vi "Main.vi"() -> ()   [LabVIEW 2014]
doc: "Use this template to build a simple state machine design pattern. Each state executes code and determines which state to transition to."
uses:
  controls/State.ctl
  controls/Data.ctl
  <vilib>/vision/Image Controls.llb/IMAQ Image.ctl
  <vilib>/userdefined/High Color/IMAQdx.ctl
panel:
  out "Tab Control":T1(tab)
  in  "Angle X":dbl(slide) scale=-90.0..90.0
  in  "Angle Y":dbl(slide) scale=-90.0..90.0
  in  "OK Button":bool
  in  "polar attributes":T2={"maximum"=1000.0, "minimum"=0.0, "clip to min"=FALSE, "log?(F)"=FALSE, "grid color"=0, "plot color"=65280, "fmt and prec"={"format"=enum."Decimal", "precision"=0}, "visible section"=8} {"minimum" format="%0.2f"; "maximum" format="%0.2f"}
  out "Image":T3(plugin-control)
  in  "Camera":refnum<k21>="cam1" caption="IMAQdx Session"
  in  "LIDAR VISA":refnum<visa-resource-name>="COM3"
  out "Data Aquired":picture
  in  "Debug Robot":bool
  in  "Reinitialize Robot":bool
  in  "Find Target":bool
  in  "Find Hole":bool
  in  "Exit":bool
  in  "Debug Angle X":dbl(slide) scale=-90.0..90.0
  in  "Debug Angle Y":dbl(slide) scale=-90.0..90.0
  in  "Debug Ok?":bool
  in  "Debug polar atributes":T2={"maximum"=300000.0, "minimum"=0.0, "clip to min"=FALSE, "log?(F)"=FALSE, "grid color"=0, "plot color"=65280, "fmt and prec"={"format"=enum."Decimal", "precision"=0}, "visible section"=8} {"minimum" format="%0.2f"; "maximum" format="%0.2f"}
  out "Debug Camera Image":T3(plugin-control)
  out "Data Aquired 2":picture
  # "Test Bench for Camera Image"
  # "Device Attributes"
  # "Select ok when all sensors and \nactuators are confirmed to be \nworking"
  # "Test Bench for Phidget Servos"
  # "Test Bench for LIDAR Data"
  # "Polar Plot Settings"
  # "Test Bench for Camera Image"
  # "Select ok when all sensors and \nactuators are confirmed to be \nworking"
  # "Test Bench for Phidget Servos"
  # "Test Bench for LIDAR Data"
  # "Polar Plot Settings"
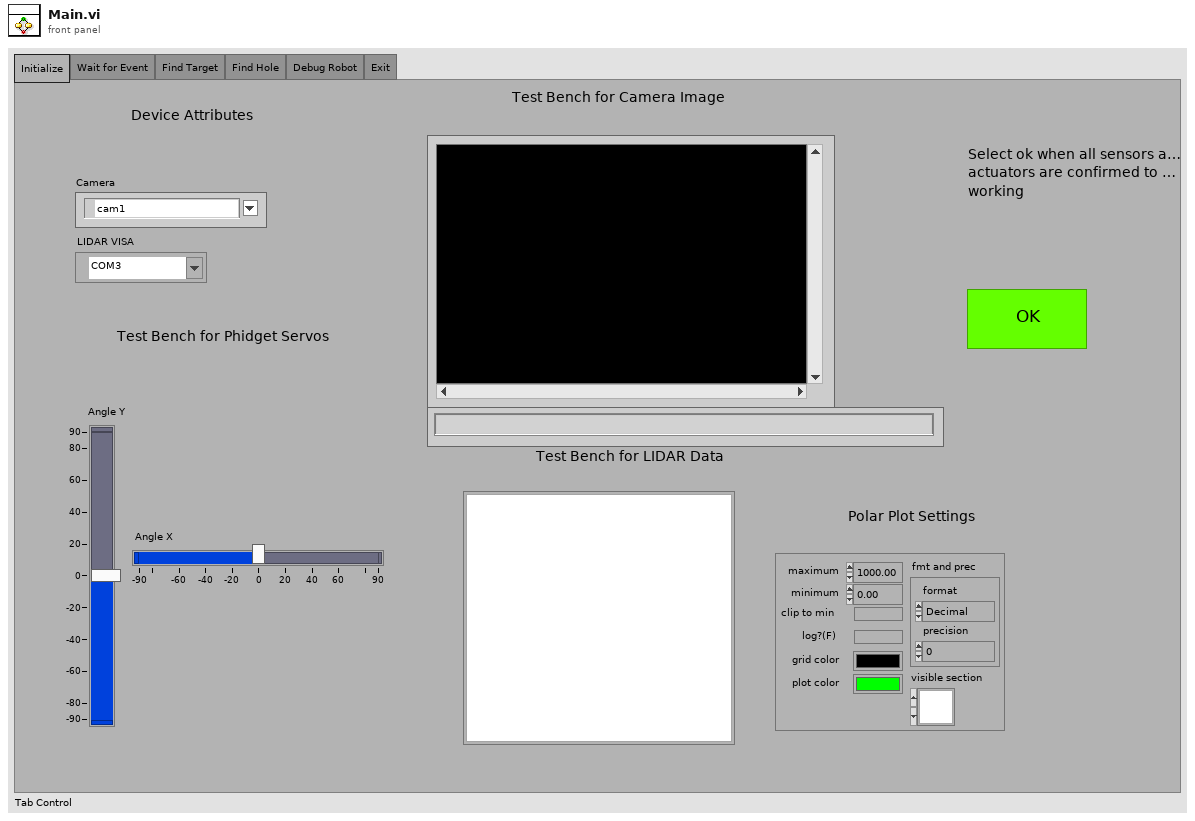
[diagram p1: front panel]
types:
  T1 = enum32{"Initialize", "Wait for Event", "Find Target", "Find Hole", "Debug Robot", "Exit"}
  T2 = cluster{"maximum":dbl, "minimum":dbl, "clip to min":bool, "log?(F)":bool, "grid color":u32, "plot color":u32, "fmt and prec":cluster{"format":enum8{"Decimal", "Scientific", "Engineering", "Binary", "Octal", "Hex"}, "precision":u8}, "visible section":u16}
  T3 = typedef "IMAQ Image.ctl" = refnum<image>
  T4 = typedef "Data.ctl" = cluster{"New Image":T3, "Session Out":T5, "LIDAR VISA Name":refnum<visa-resource-name>, "Phidget Device Out":i32, "Lidar Data":cluster{dbl, dbl}[], "polar attributes":cluster{"maximum":dbl, "minimum":dbl, "clip to min":bool, "log?(F)":bool, "grid color":u32, "plot color":u32, "fmt and prec":cluster{"format":enum8{"Decimal", "Scientific", "Engineering", "Binary", "Octal", "Hex"}, "precision":u8}, "visible section":u16}, "Debug Statement":string, "Servo Angles":cluster{"Angle X":dbl, "Angle Y":dbl}}
  T5 = typedef "IMAQdx.ctl" = refnum<k21>
  T6 = typedef "State.ctl" = enum16{"Initialize", "Wait for Event", "Find Target", "Find Hole", "Debug Robot", "Exit"}
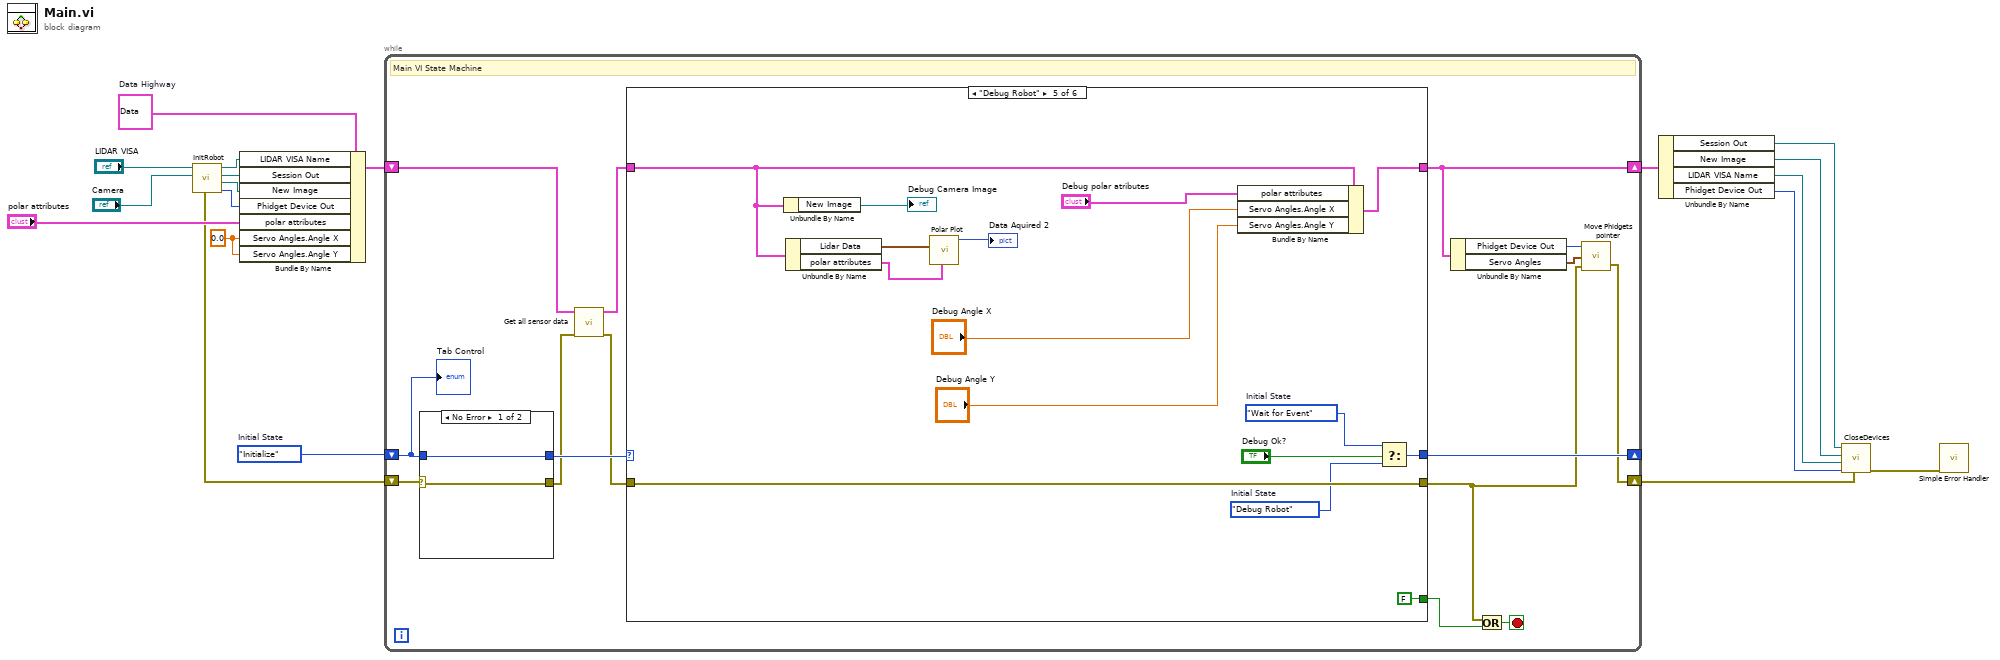
[diagram p0: block diagram]
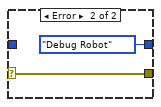
[diagram p2: hidden frame]
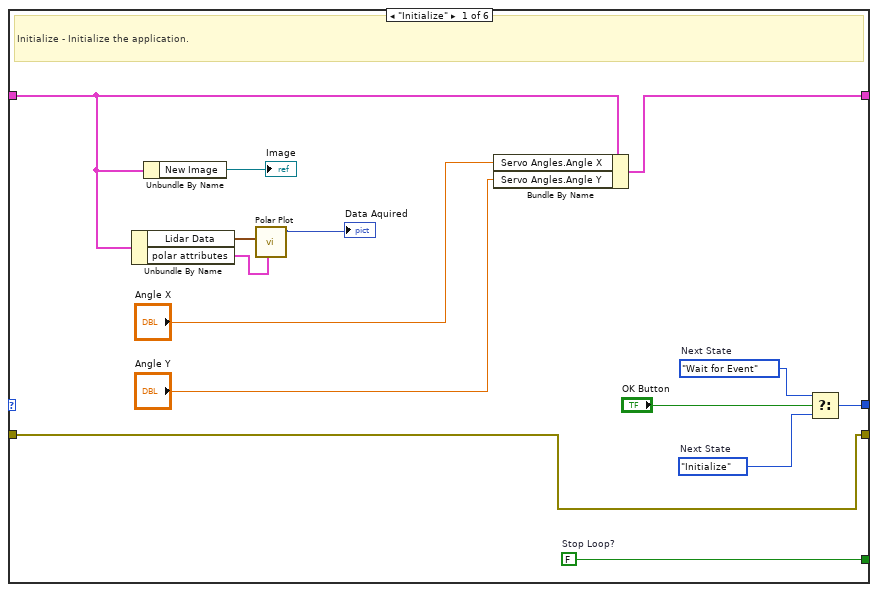
[diagram p3: hidden frame]
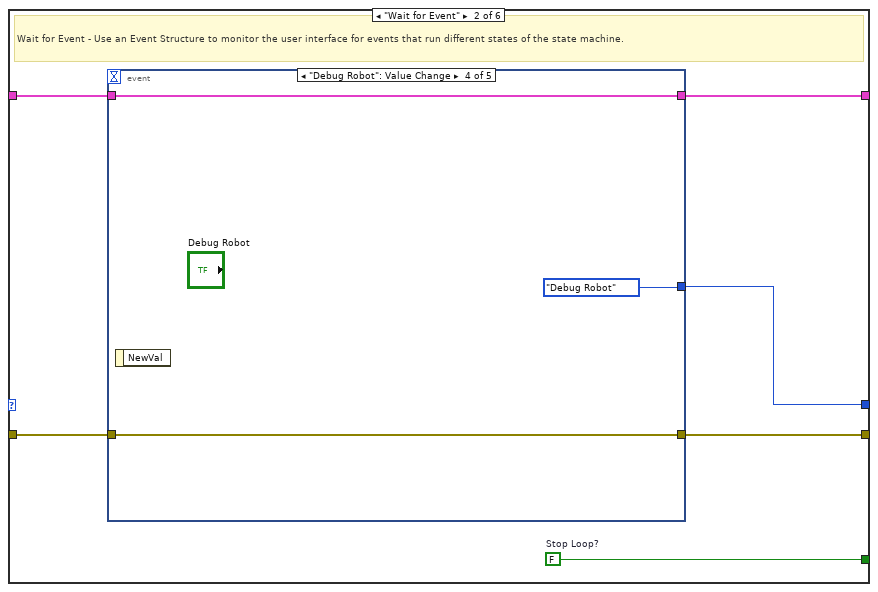
[diagram p4: hidden frame]
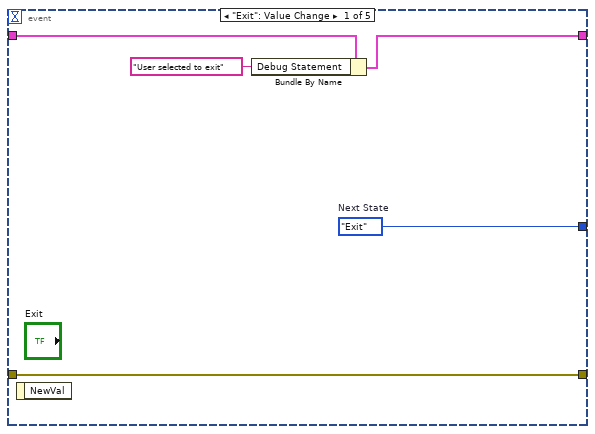
[diagram p5: hidden frame]
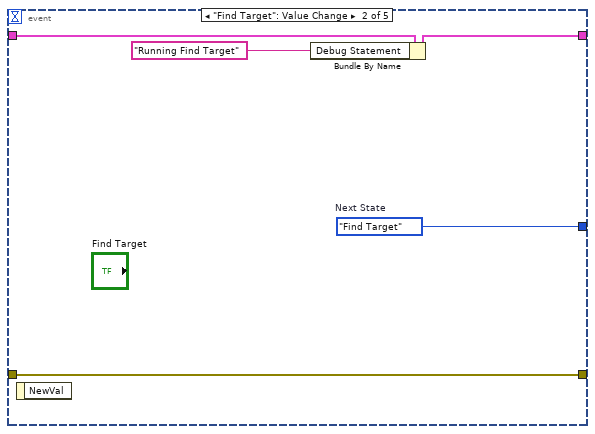
[diagram p6: hidden frame]
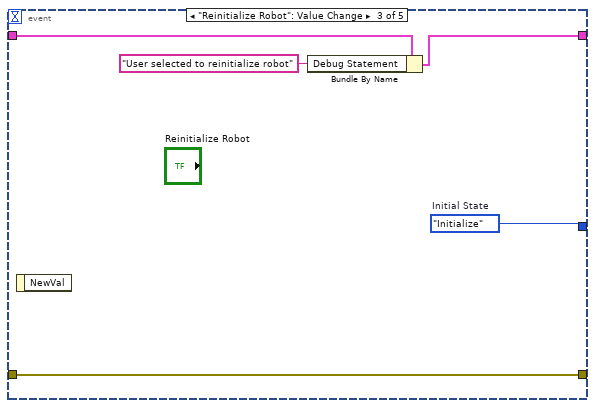
[diagram p7: hidden frame]
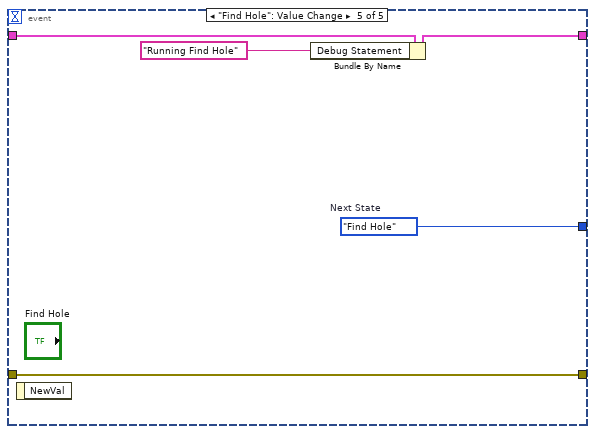
[diagram p8: hidden frame]
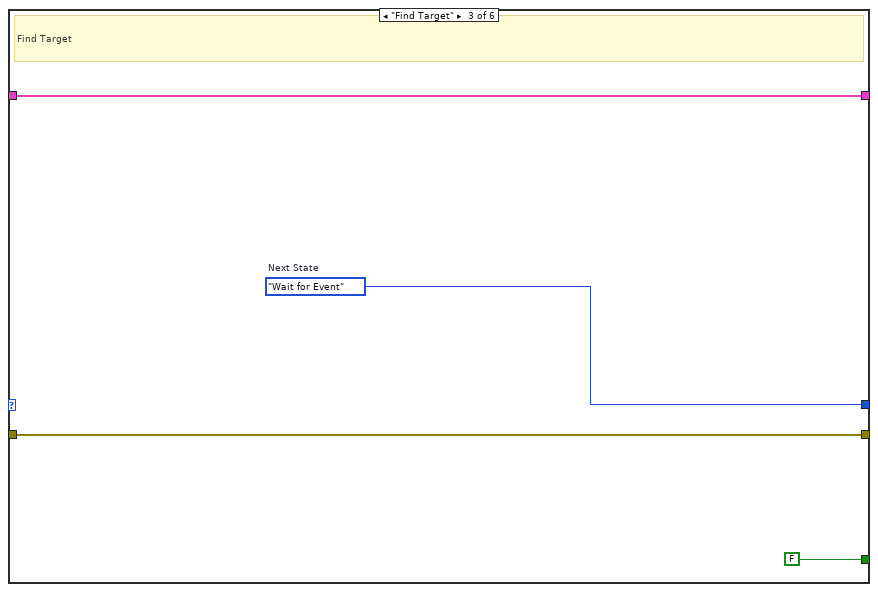
[diagram p9: hidden frame]
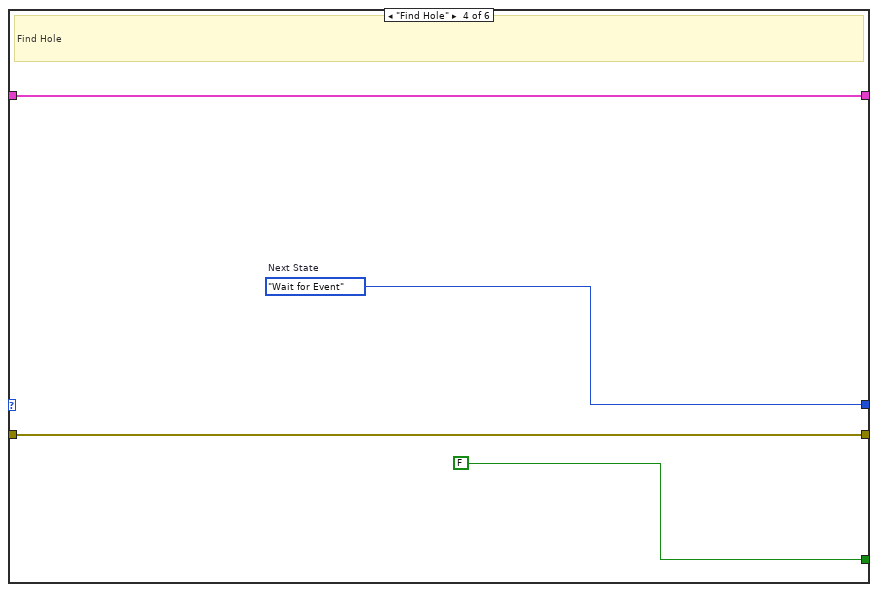
[diagram p10: hidden frame]
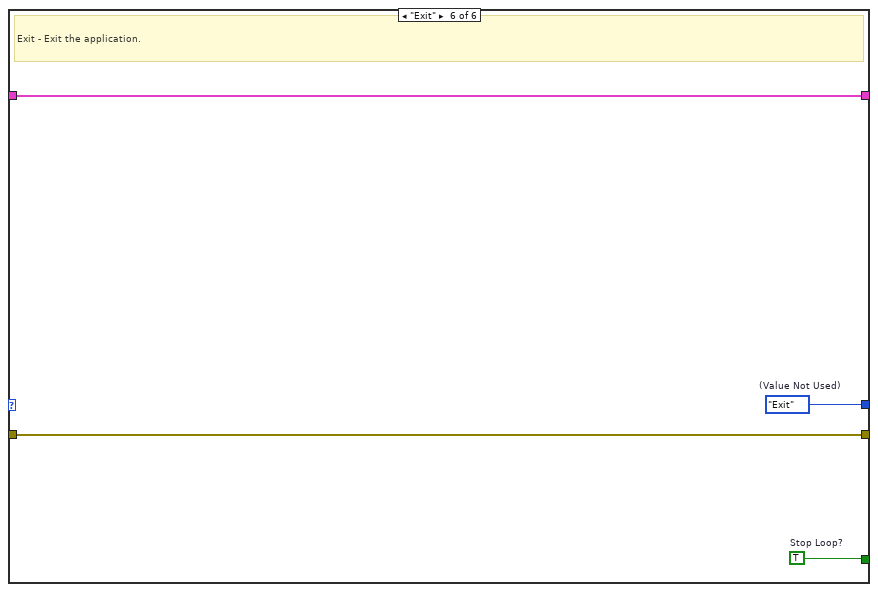
[diagram p11: hidden frame]
diagram:
  w1 = 0.0 ("Servo Angles.Angle X")
  w18 = T4 {"New Image"=refnum, "Session Out"="", "LIDAR VISA Name"="", "Phidget Device Out"=0, "Lidar Data"=[], "polar attributes"={"maximum"=0.0, "minimum"=0.0, "clip to min"=FALSE, "log?(F)"=FALSE, "grid color"=6710886, "plot color"=65280, "fmt and prec"={"format"=enum."Decimal", "precision"=0}, "visible section"=8}, "Debug Statement"="", "Servo Angles"={"Angle X"=0.0, "Angle Y"=0.0}}  # Data Highway
  w19 = State."Initialize"  # Initial State
  n1 = call "InitRobot.vi"("Camera Name"="Camera", "VISA resource name"="LIDAR VISA") -> ("Device Out"=w10:i32, "New Image"=w11:T3, "Session Out"=w12:T5, "VISA resource name out"=w13:refnum<visa-resource-name>, "error out"=w9:errorcluster)  [unwired: 4 in]
  n2 = Bundle By Name(cluster=w18, "LIDAR VISA Name"=w13, "Session Out"=w12, "New Image"=w11, "Phidget Device Out"=w10, "polar attributes"="polar attributes", "Servo Angles.Angle X"=w1, "Servo Angles.Angle Y"=w1) -> (w17:T4)
  n3 = while {
    shift-right: [w34] -> _
    shift-left: w19 -> [w29]
    shift-right: [w24] -> w6
    shift-left: w17 -> [w28]
    shift-right: [w21] -> w8
    shift-left: w9 -> [w31]
    stop <- w32 stop-if-true
    # "Main VI State Machine"
    n4 = case shown="No Error" w31 {
      selector: w31 -> [w35 w37]
      tunnel: [w36 State."Debug Robot" ("Initial State")] -> w30
      tunnel: w29 -> [w36 _]
      tunnel: [w35 w37] -> w26
      frame No Error {
      }
      frame Error {
      }
    }
    n5 = call "Get all sensor data.vi"("error in"=w26, "Data Highway In"=w28) -> ("error out"=w25:errorcluster, "Data Highway Out"=w27:T4)  [unwired: 6 in]
    n6 = case shown="\"Debug Robot\"" w30 {
      tunnel: [w51 w58 w85 w89 w93 w105] -> w34
      tunnel: [w52 w57 FALSE ("Stop Loop?") FALSE ("Stop Loop?") FALSE ("Stop Loop?") w106] -> w33
      tunnel: w27 -> [w42 w56 w83 w87 w95 w108]
      tunnel: [w41 w55 w83 w87 w94 w108] -> w24
      tunnel: w25 -> [w46 w54 w82 w86 w104 w107]
      tunnel: [w46 w53 w82 w86 w104 w107] -> w22
      frame "Initialize" {
        w48 = State."Initialize"  # Next State
        w52 = FALSE  # Stop Loop?
        w49 = State."Wait for Event"  # Next State
        # "Initialize - Initialize the application."
        n7 = Unbundle By Name(w42) -> ("Lidar Data"=w45:cluster{dbl, dbl}[], "polar attributes"=w44:T2)
        n8 = Unbundle By Name(w42) -> ("New Image"=→"Image":T3)
        n9 = call <vilib>:"Polar Plot.vi"("polar attributes"=w44, "data array [mag, phase (deg)]"=w45) -> ("new picture"=→"Data Aquired":picture)  [unwired: 9 in]
        n10 = Bundle By Name(cluster=w42, "Servo Angles.Angle X"="Angle X", "Servo Angles.Angle Y"="Angle Y") -> (w41:T4)
        n11 = Select(t=w49, s="OK Button", f=w48) -> (s? t:f=w51:T6)
      }
      frame "Wait for Event" {
        w57 = FALSE  # Stop Loop?
        # "Wait for Event - Use an Event Structure to monitor the user interface for events that run different states of the state machine."
        n12 = event shown="[3] \"Debug Robot\": Value Change" {
          selector: _ -> [_ _ _ _ _]
          dyn-events: _ -> [_ _ _ _ _]
          timeout: _ -> [_ _ _ _ _]
          tunnel: [w63 w68 w72 State."Debug Robot" ("Initial State") w81] -> w58
          tunnel: w56 -> [w61 w67 w71 w76 w80]
          tunnel: [w60 w66 w70 w76 w79] -> w55
          tunnel: w54 -> [w62 w65 w73 w75 w78]
          tunnel: [w62 w65 w73 w75 w78] -> w53
          event "Exit": Value Change {
            w63 = State."Exit"  # Next State
            n13 = event-data() -> ()  [unwired: 1 in, 1 out]
            n14 = Bundle By Name(cluster=w61, "Debug Statement"="User selected to exit") -> (w60:T4)
          }
          event "Find Target": Value Change {
            w68 = State."Find Target"  # Next State
            n15 = event-data() -> ()  [unwired: 1 in, 1 out]
            n16 = Bundle By Name(cluster=w67, "Debug Statement"="Running Find Target" ("Running User State 1")) -> (w66:T4)
          }
          event "Reinitialize Robot": Value Change {
            w72 = State."Initialize"  # Initial State
            n17 = event-data() -> ()  [unwired: 1 in, 1 out]
            n18 = Bundle By Name(cluster=w71, "Debug Statement"="User selected to reinitialize robot") -> (w70:T4)
          }
          event "Debug Robot": Value Change {
            n19 = event-data() -> ()  [unwired: 1 in, 1 out]
          }
          event "Find Hole": Value Change {
            w81 = State."Find Hole"  # Next State
            n20 = event-data() -> ()  [unwired: 1 in, 1 out]
            n21 = Bundle By Name(cluster=w80, "Debug Statement"="Running Find Hole" ("Running User State 2")) -> (w79:T4)
          }
        }
      }
      frame "Find Target" {
        w85 = State."Wait for Event"  # Next State
        # "Find Target"
      }
      frame "Find Hole" {
        w89 = State."Wait for Event"  # Next State
        # "Find Hole"
      }
      frame "Debug Robot" {
        w91 = State."Debug Robot"  # Initial State
        w92 = State."Wait for Event"  # Initial State
        n22 = Unbundle By Name(w95) -> ("New Image"=→"Debug Camera Image":T3)
        n23 = Unbundle By Name(w95) -> ("Lidar Data"=w101:cluster{dbl, dbl}[], "polar attributes"=w100:T2)
        n24 = call <vilib>:"Polar Plot.vi"("polar attributes"=w100, "data array [mag, phase (deg)]"=w101) -> ("new picture"=→"Data Aquired 2":picture)  [unwired: 9 in]
        n25 = Bundle By Name(cluster=w95, "polar attributes"="Debug polar atributes", "Servo Angles.Angle X"="Debug Angle X", "Servo Angles.Angle Y"="Debug Angle Y") -> (w94:T4)
        n26 = Select(t=w92, s="Debug Ok?", f=w91) -> (s? t:f=w93:T6)
      }
      frame "Exit" {
        w106 = TRUE  # Stop Loop?
        w105 = State."Exit"  # (Value Not Used)
        # "Exit - Exit the application."
      }
    }
    n27 = Unbundle By Name(w24) -> ("Phidget Device Out"=w23:i32, "Servo Angles"=w20:cluster{"Angle X":dbl, "Angle Y":dbl})
    n28 = Or(x=w22, y=w33) -> (x .or. y?=w32:bool)
    n29 = call "Move Phidgets pointer.vi"("error in (no error)"=w22, "Servo Angles"=w20, "Device In"=w23) -> ("error out"=w21:errorcluster)  [unwired: 1 out]
    "Tab Control" <- w29
  }
  n30 = Unbundle By Name(w6) -> ("Session Out"=w5:T5, "New Image"=w4:T3, "LIDAR VISA Name"=w3:refnum<visa-resource-name>, "Phidget Device Out"=w2:i32)
  n31 = call "CloseDevices.vi"("error in"=w8, "Device In"=w2, "VISA resource name"=w3, "Image"=w4, "Session In"=w5) -> ("error out"=w7:errorcluster)  [unwired: 6 in]
  n32 = call <vilib>:"Simple Error Handler.vi"("error in (no error)"=w7) -> ()  [unwired: 4 in, 5 out]
